vi "Read lockin time constant.vi"() -> (2 "time constant":dbl[unit])   [LabVIEW 2009, in "Lockin.lvclass"]
doc: "Reads the current time constant from the lock-in detector."
uses:
  Lockin.lvclass
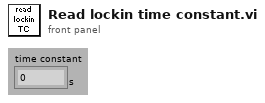
[diagram p1: front panel]
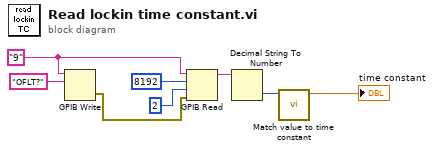
[diagram p0: block diagram]
diagram:
  w7 = "9" ("address string")
  n1 = GPIB Write(0:w7, 1:"OFLT?" ("data")) -> (6:w4:errorcluster)  [unwired: 1 in, 3 out]
  n2 = GPIB Read(0:w7, 1:8192 ("byte count"), 2:i16 2 ("mode (0)"), 3:w4) -> (5:w3:string)  [unwired: 3 out]
  n3 = Decimal String To Number(string=w3) -> (number=w2:i32)  [unwired: 3 out]
  n4 = call "Match value to time constant.vi"("integer"=w2) -> ("time constant"=→"time constant":dbl[unit])  [unwired: 10 out]
